vi "Add Package.vi"(8 "error in (no error)":errorcluster, 10 "Package":refnum<class "Package.lvclass">, 11 "Coverage in":refnum<class "Coverage.lvclass">) -> (0 "error out":errorcluster, 3 "Coverage out":refnum<class "Coverage.lvclass">)   [LabVIEW 2017, in "Cobertura.lvlib" / "Coverage.lvclass"]
uses:
  Coverage.lvclass
  Package/Package.lvclass
  Coverage.lvclass/Coverage.ctl
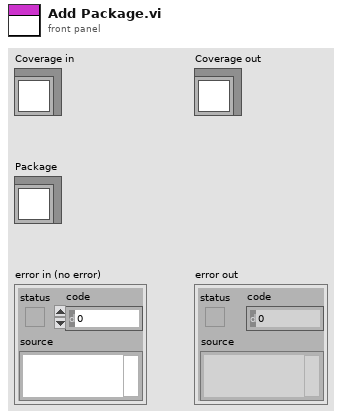
[diagram p1: front panel]
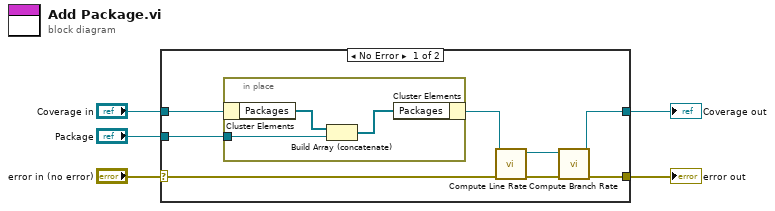
[diagram p0: block diagram]
diagram:
  n1 = case shown="No Error" "error in (no error)" {
    selector: "error in (no error)" -> [w13 w18]
    tunnel: [w8 w18] -> w2
    tunnel: [w6 w17] -> w4
    tunnel: "Coverage in" -> [w12 w17]
    tunnel: "Package" -> [w11 _]
    frame No Error {
      n2 = in-place {
        in-place-border: w11 -> [w14]
        n3 = in-place-cluster #1(w12) -> ("Packages"=w16:refnum<class "Package.lvclass">[])
        n4 = Build Array (concatenate)(w16, w14) -> (w15:refnum<class "Package.lvclass">[])
        n5 = in-place-cluster #1("Packages"=w15) -> (w9:refnum<class "Coverage.lvclass">)
      }
      n6 = call "Compute Line Rate.vi"("error in (no error)"=w13, "Coverage in"=w9) -> ("error out"=w10:errorcluster, "Coverage out"=w7:refnum<class "Coverage.lvclass">)  [unwired: 8 in]
      n7 = call "Compute Branch Rate.vi"("error in (no error)"=w10, "Coverage in"=w7) -> ("error out"=w8:errorcluster, "Coverage out"=w6:refnum<class "Coverage.lvclass">)  [unwired: 8 in]
    }
    frame Error {
    }
  }
  "error out" <- w2
  "Coverage out" <- w4
